vi "RFID Write Example.vi"() -> ()   [LabVIEW 2012, in "Phidget RFID.lvlib"]
uses:
  <instrlib>/Phidgets/Phidget RFID/Phidget RFID.lvlib
  <instrlib>/Phidgets/Phidget RFID/Public/RFIDStart.vi
  <instrlib>/Phidgets/Phidget RFID/Public/RFIDClose.vi
  <instrlib>/Phidgets/Phidget Common/Phidget Common.lvlib
panel:
  in  "Lock":bool
  in  "string":string
  in  "protocol":i32(ring) items=["PROTOCOL_EM4100"=1, "PROTOCOL_ISO11785_FDX_B"=2, "PROTOCOL_PHIDGETS"=3]
  out "error out":errorcluster
  in  "error in (no error)":errorcluster
  in  "Device Info":T1={"Serial Number"=-1, "Channel"=0, "Port"=0}
  out "Attached?":bool
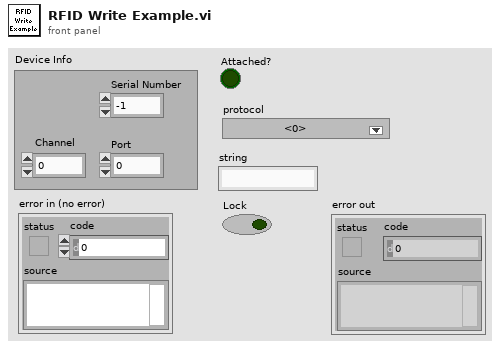
[diagram p1: front panel]
types:
  T1 = cluster{"Serial Number":i32, "Channel":i32, "Port":i32}
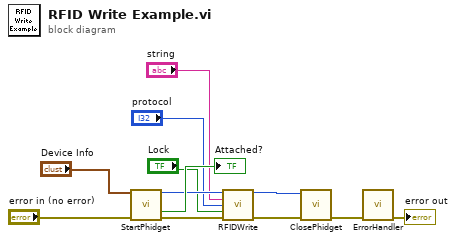
[diagram p0: block diagram]
diagram:
  n1 = call-poly <instrlib>:"StartPhidget.vi"("Device Info"="Device Info", "error in (no error)"="error in (no error)") -> ("Phidget ID"=w7:u64, "Attached?"=→"Attached?":bool, "error out"=w6:errorcluster)  [unwired: 10 in, 1 out]
  n2 = call <instrlib>:"RFIDWrite.vi"("Device In"=w7, "string"="string", "protocol"="protocol", "Lock"="Lock", "error in (no error)"=w6) -> ("Device Out"=w4:u64, "error out"=w5:errorcluster)  [unwired: 9 in]
  n3 = call-poly <instrlib>:"ClosePhidget.vi"("error in"=w5, "Device In"=w4) -> ("error out"=w9:errorcluster)  [unwired: 9 in]
  n4 = call <instrlib>:"ErrorHandler.vi"("error in"=w9) -> ("error out"=→"error out":errorcluster)  [unwired: 9 in, 1 out]
